vi "XGB 개별 읽기.vi"() -> ()   [LabVIEW 2014]
uses:
  <vilib>/Instr/_visa.llb/VISA Configure Serial Port (Instr).vi
panel:
  in  "VISA resource name":refnum<visa-resource-name>="COM13"
  out "error out":errorcluster={"status"=FALSE, "code"=1073676294, "source"="XGB 읽기.vi 안에 VISA 읽기"} caption="에러 출력"
  out "응답 프레임":string="\u000600RSB016430313233323330303233303032333030323330303233303000000000000000000000000000000000000000000000000000000000000000000000000000000000000000000000000000000000000000000000000000000000000000000000000000000000\u0003"
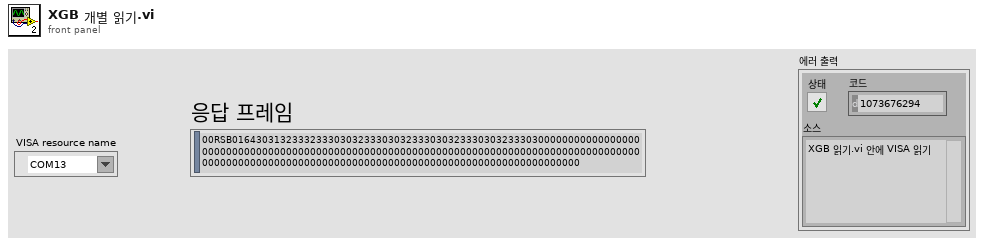
[diagram p1: front panel]
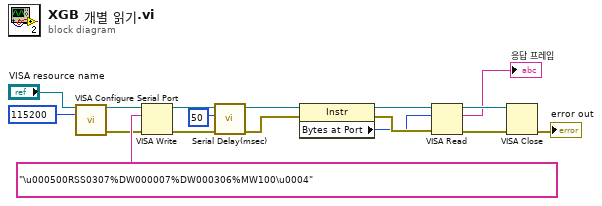
[diagram p0: block diagram]
diagram:
  n1 = call-poly "VISA Configure Serial Port"("VISA resource name"="VISA resource name", "baud rate (9600)"=u32 115200 ("baud rate")) -> ("VISA resource name out"=w7:refnum<visa-resource-name>, "error out"=w6:errorcluster)  [unwired: 12 in]
  n2 = VISA Write(VISA resource name=w7, write buffer="\u000500RSS0307%DW000007%DW000306%MW100\u0004" ("요구 프레임"), error in (no error)=w6) -> (VISA resource name out=w14:refnum<visa-resource-name>, error out=w11:errorcluster)  [unwired: 1 out]
  n3 = call "Serial Delay(msec).vi"("에러 입력(에러 없음)"=w11, "milliseconds to wait"=u32 50, "VISA 참조 번호 입력"=w14) -> ("에러 출력"=w12:errorcluster, "VISA 참조 번호 출력"=w13:refnum<visa-resource-name>)  [unwired: 7 in]
  n4 = property class="Instr"(reference=w13, error in=w12) -> (reference out=w15:refnum<visa-resource-name>, error out=w16:errorcluster, "Bytes at Port"=w1:u32)
  n5 = VISA Read(VISA resource name=w15, byte count=w1, error in (no error)=w16) -> (VISA resource name out=w5:refnum<visa-resource-name>, read buffer=→"응답 프레임":string, error out=w4:errorcluster)  [unwired: 1 out]
  n6 = VISA Close(VISA resource name=w5, error in (no error)=w4) -> (error out=→"error out":errorcluster)
